vi "Log Squence Save.vi"(8 "Fehler (in)":errorcluster caption="Fehlerkonstante", 9 "Item Names":string[](array[string]), 11 "Aktuelle Gasliste gesamt":T1[](array[typedef])) -> (0 "Fehler (out)":errorcluster caption="Fehlerkonstante")   [LabVIEW 2020, in "LogKonfig.lvlib"]
uses:
  Visualisierungs Elemente/String - Ausgabefeld.ctl
  Log Sequence FGV Aktion.ctl
  LogKonfig.lvlib
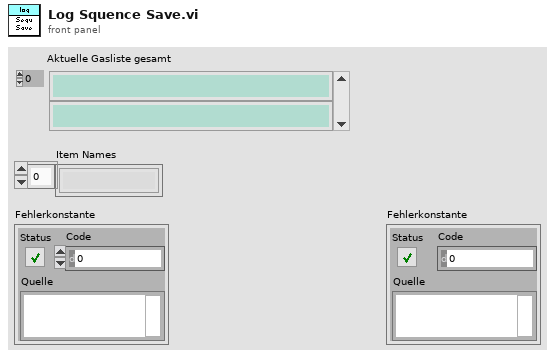
[diagram p1: front panel]
types:
  T1 = typedef "String - Ausgabefeld.ctl" = string
  T2 = typedef "LogKonfig.lvlib/Log Sequence FGV Aktion.ctl" = enum16{"initialisieren", "lesen", "schreiben", "laden", "speichern", "übertragen"}
  T3 = cluster{"Index Array":i32[], "Namen Array":string[], "Spektrum File Name":bool}
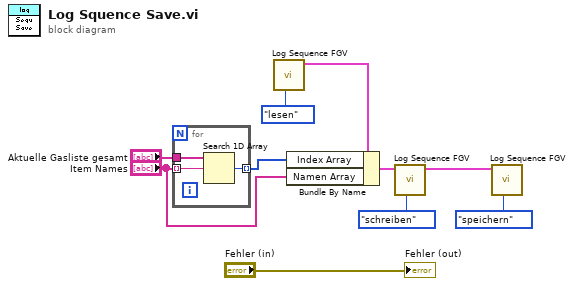
[diagram p0: block diagram]
diagram:
  n1 = for {
    tunnel: "Aktuelle Gasliste gesamt" -> [w13]
    tunnel: "Item Names" -> [w12] mode=indexing
    tunnel: [w11] -> w7 mode=indexing
    n2 = Search 1D Array(1D array=w13, element=w12) -> (index of element=w11:i32)  [unwired: 1 in]
  }
  n3 = call "Log Sequence FGV.vi"("Aktion"=Log_Sequence_FGV_Aktion."lesen") -> ("Cluster (out)"=w1:T3)  [unwired: 10 in]
  n4 = Bundle By Name(cluster=w1, "Index Array"=w7, "Namen Array"="Item Names") -> (w10:T3)
  n5 = call "Log Sequence FGV.vi"("Aktion"=Log_Sequence_FGV_Aktion."schreiben", "Cluster (in)"=w10) -> ("Cluster (out)"=w5:T3)  [unwired: 9 in]
  n6 = call "Log Sequence FGV.vi"("Aktion"=Log_Sequence_FGV_Aktion."speichern", "Cluster (in)"=w5) -> ()  [unwired: 9 in, 1 out]
  "Fehler (out)" <- "Fehler (in)"
